vi "按钮回调.vi"(4 "按钮":refnum<user-event>, 5 "事件数据":cluster{"oldValue":bool, "newValue":bool}, 6 "控件引用":refnum<k24>, 7 "事件通用数据":cluster{"事件源":i32, "事件类型":u32, "时间标识":u32}) -> ()   [LabVIEW 2018]
uses:
  data/MyControlAll.dll
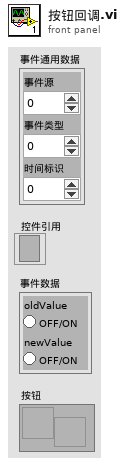
[diagram p1: front panel]
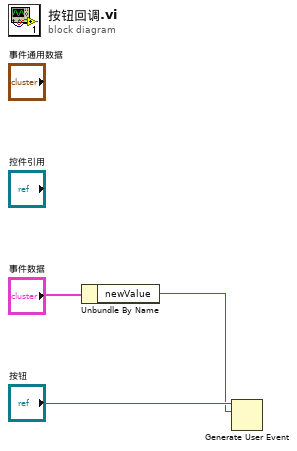
[diagram p0: block diagram]
diagram:
  n1 = Unbundle By Name("事件数据") -> ("newValue"=w1:bool)
  n2 = Generate User Event(user event="按钮", event data cluster=w1) -> ()  [unwired: 2 in, 2 out]
